vi "RT Main - No FPGA (IMAQ).vi"() -> ()   [LabVIEW 2017]
doc: "The myRIO Custom FPGA Project template acquires button data from the onboard button and displays the button value on a Boolean indicator. The SYS.RDY indicator shows the FPGA status."
uses:
  SoC IP Library/Controls/Image Size.ctl
  <vilib>/userdefined/High Color/IMAQdx.ctl
  SoC IP Library/SoC IP Library.lvlib
  <vilib>/vision/driver/NI_Vision_Acquisition_Software.lvlib
  <vilib>/vision/NI_Vision_Development_Module.lvlib
panel:
  in  "Display?":bool
  out "Image Out":T1(plugin-control)
  out "Image In":T1(plugin-control)
  in  "Live":bool
  out "FPS":u32
  out "error out":errorcluster
  in  "Stop":bool
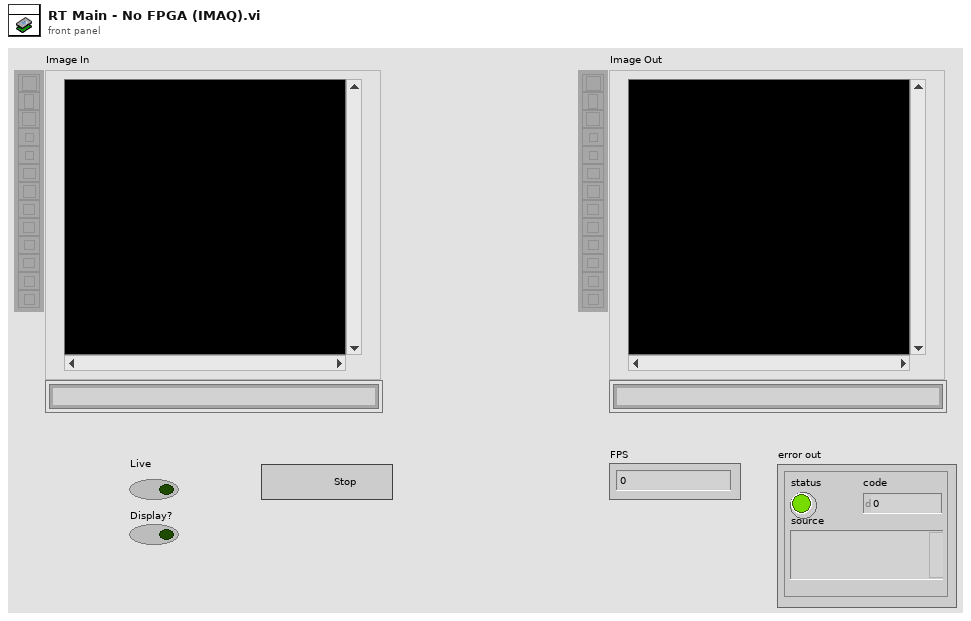
[diagram p1: front panel]
types:
  T1 = typedef "IMAQ Image.ctl" = refnum<image>
  T2 = typedef "IMAQdx.ctl" = refnum<k21>
  T3 = typedef "SoC IP Library.lvlib/Image Size.ctl" = cluster{"Rows (X)":u16, "Colums (Y)":u16}
  T4 = typedef "Image Type" = u32
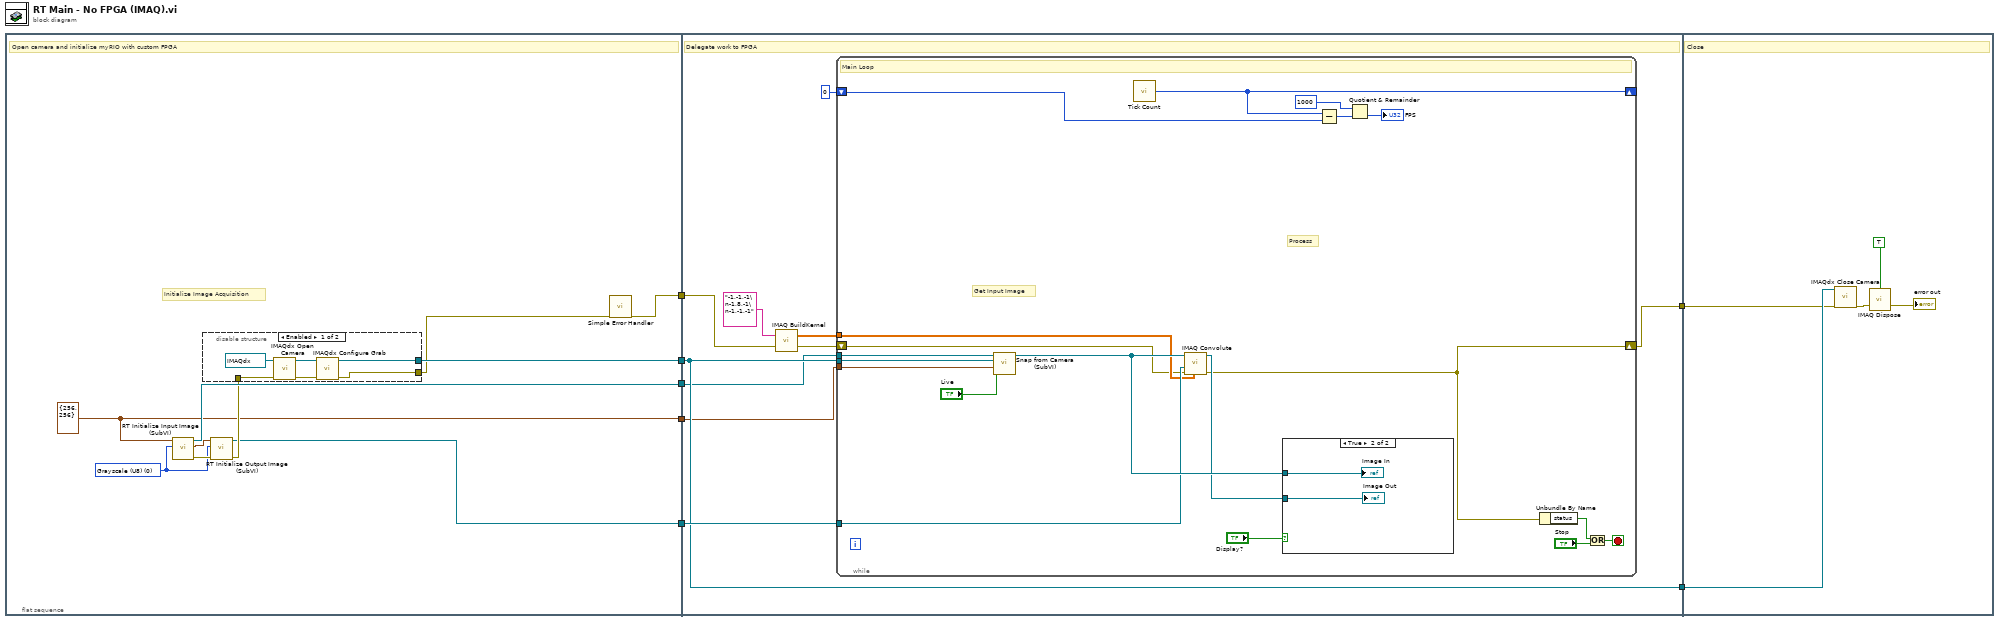
[diagram p0: block diagram]
diagram:
  n1 = flat-sequence {
    tunnel: [w12] -> w7
    tunnel: [w17] -> w6
    tunnel: [w16] -> w5
    tunnel: [w10] -> w4
    tunnel: [w9] -> w2
    tunnel: w7 -> [w33]
    tunnel: w6 -> [w32]
    tunnel: w5 -> [w31]
    tunnel: w4 -> [w29]
    tunnel: [w32] -> w3
    tunnel: w2 -> [w30]
    tunnel: [w25] -> w1
    tunnel: w3 -> [w57]
    tunnel: w1 -> [w56]
    frame #0 {
      w9 = T3 {"Rows (X)"=256, "Colums (Y)"=256} ("Image Size")
      w13 = T4 0 items=["Grayscale (U8)", "Grayscale (I16)", "Grayscale (SGL)", "Complex (CSG)", "RGB (U32)", "HSL (U32)", "RGB (U64)", "Grayscale (U16)"] ("Image Type")
      # "Initialize Image Acquisition"
      # "Open camera and initialize myRIO with custom FPGA"
      n2 = call "RT Initialize Input Image (SubVI).vi"("Image Type"=w13, "Image Size In"=w9) -> ("error out"=w15:errorcluster, "Input Image Size Out"=w11:T3, "Input Image Out"=w16:T1)  [unwired: 7 in]
      n3 = call "RT Initialize Output Image (SubVI).vi"("error in (no error)"=w15, "Image Type"=w13, "Image Size In"=w11) -> ("error out"=w14:errorcluster, "Output Image Out"=w12:T1)  [unwired: 7 in]
      n4 = disable-structure shown="Enabled" {
        disable-tunnel: [w20 _] -> w17
        disable-tunnel: w14 -> [w19 w24]
        disable-tunnel: [w18 w24] -> w8
        frame Enabled {
          n5 = call <vilib>:"IMAQdx Open Camera.vi"("error in"=w19, "Session In"=T2 "cam0") -> ("error out"=w22:errorcluster, "Session Out"=w21:T2)  [unwired: 8 in]
          n6 = call <vilib>:"IMAQdx Configure Grab.vi"("error in"=w22, "Session In"=w21) -> ("error out"=w18:errorcluster, "Session Out"=w20:T2)  [unwired: 8 in]
        }
        frame Disabled {
        }
      }
      n7 = call <vilib>:"Simple Error Handler.vi"("error in (no error)"=w8) -> ("error out"=w10:errorcluster)  [unwired: 4 in, 4 out]
    }
    frame #1 {
      # "Delegate work to FPGA"
      n8 = call "IMAQ BuildKernel"("Kernel String"="-1,-1,-1\n-1,8,-1\n-1,-1,-1", "error in (no error)"=w29) -> ("Kernel"=w27:sgl[][], "error out"=w26:errorcluster)  [unwired: 3 in]
      n9 = while {
        shift-right: [w51] -> _
        shift-left: u32 0 ("Tick Count(mSec)") -> [w50]
        tunnel: w32 -> [w49]
        tunnel: w33 -> [w39]
        tunnel: w31 -> [w48]
        tunnel: w30 -> [w45]
        tunnel: w27 -> [w38]
        shift-right: [w35] -> w25
        shift-left: w26 -> [w36]
        stop <- w52 stop-if-true
        # "Process"
        # "Get Input Image"
        # "Main Loop"
        n10 = call "Snap from Camera (SubVI).vi"("Live"="Live", "Image Size in"=w45, "Session In"=w49, "Image in"=w48) -> ("Image out"=w40:T1)  [unwired: 3 in, 4 out]
        n11 = call "Tick Count"() -> ("Tick Count(mSec)"=w51:u32)
        n12 = call "IMAQ Convolute"("Kernel"=w38, "error in (no error)"=w36, "Image Dst"=w39, "Image Src"=w40) -> ("error out"=w35:errorcluster, "Image Dst Out"=w37:T1)  [unwired: 6 in]
        n13 = case shown="True" "Display?" {
          tunnel: w40 -> [_ w55]
          tunnel: w37 -> [_ w54]
          frame False {
          }
          frame True {
            "Image In" <- w55
            "Image Out" <- w54
          }
        }
        n14 = Subtract(x=w51, y=w50) -> (x-y=w42:u32)
        n15 = Quotient & Remainder(x=u32 1000, y=w42) -> (floor(x/y)=→"FPS":u32)  [unwired: 1 out]
        n16 = Unbundle By Name(w35) -> ("status"=w44:bool)
        n17 = Or(x=w44, y="Stop") -> (x .or. y?=w52:bool)
      }
    }
    frame #2 {
      # "Close"
      n18 = call <vilib>:"IMAQdx Close Camera.vi"("error in"=w56, "Session In"=w57) -> ("error out"=w58:errorcluster)  [unwired: 9 in]
      n19 = call "IMAQ Dispose"("All Images? (No)"=TRUE, "error in (no error)"=w58) -> ("error out"=→"error out":errorcluster)  [unwired: 4 in]
    }
  }
